vi "SelectCamera.vi"() -> (2 "error out":errorcluster, 3 "Refnum out":T1)   [LabVIEW 2017]
uses:
  <vilib>/userdefined/High Color/IMAQdx.ctl
panel:
  in  "Select Control":T1
  in  "stop":bool
  # "Select Camera"
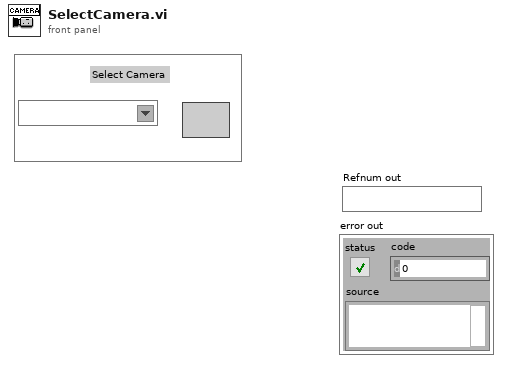
[diagram p1: front panel]
types:
  T1 = typedef "IMAQdx.ctl" = refnum<k21>
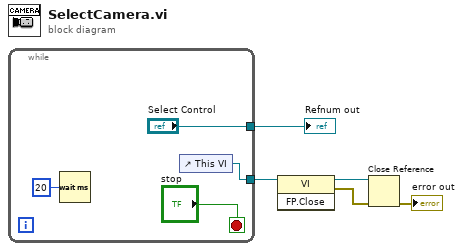
[diagram p0: block diagram]
diagram:
  n1 = while {
    tunnel: ["Select Control"] -> w5
    tunnel: [w6] -> w4
    stop <- "stop" stop-if-true
    n2 = Wait (ms)(milliseconds to wait=u32 20) -> ()  [unwired: 1 out]
    n3 = control-ref of="This VI"() -> (w6:refnum<vi>)
  }
  "Refnum out" <- w5
  n4 = invoke class="VI" method="FP.Close"(reference=w4) -> (reference out=w3:refnum<vi>, error out=w2:errorcluster)  [unwired: 2 in, 1 out]
  n5 = Close Reference(reference=w3, error in (no error)=w2) -> (error out=→"error out":errorcluster)
